vi "Configure Multi Eval Meas List Segment DMRS Type A.vi"(0 "VISA resource name":refnum<visa-resource-name>, 1 "BWP (0)":i32, 2 "Additional Position (0)":i32, 5 "Instance (1)":T2=1, 7 "Segment (1)":i32=1, 9 "CC (1)":T1=1, 11 "error in (no error)":errorcluster, 12 "Config Type (1)":i32=1, 13 "Max Length (1)":i32=1) -> (4 "VISA resource name out":refnum<visa-resource-name>, 15 "error out":errorcluster)   [LabVIEW 2020, in "Rohde&Schwarz CMWXP NR FR1 Measurement.lvlib"]
doc: "Configures the DM-RS for mapping type A. The settings apply to the <BWP> on carrier <cc> in segment <no>.\n\nAttribute:\nRSCMWXPNRFR1M_ATTR_MULTI_EVAL_MEAS_LIST_SEGMENT_DMRS_TYPE_A\n\nRemote-control command:\nCONFigure:NRSub:MEAS<i>:LIST:SEGMent<no>[:CC<cc>]:BWPart:PUSCh:DMTA"
uses:
  <instrlib>/Rohde&Schwarz CMWXP NR FR1 Measurement/Rohde&Schwarz CMWXP NR FR1 Measurement.lvlib
  <instrlib>/Rohde&Schwarz CMWXP NR FR1 Measurement/Private/_Instance.ctl
  <instrlib>/Rohde&Schwarz CMWXP NR FR1 Measurement/Private/_Carrier Component.ctl
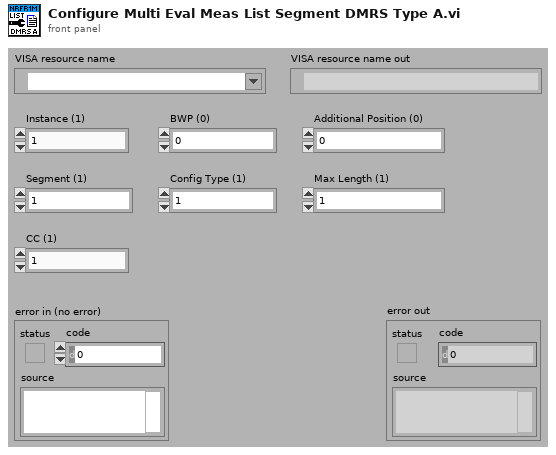
[diagram p1: front panel]
types:
  T1 = typedef "Rohde&Schwarz CMWXP NR FR1 Measurement.lvlib/_Carrier Component.ctl" = i32
  T2 = typedef "Rohde&Schwarz CMWXP NR FR1 Measurement.lvlib/_Instance.ctl" = i32
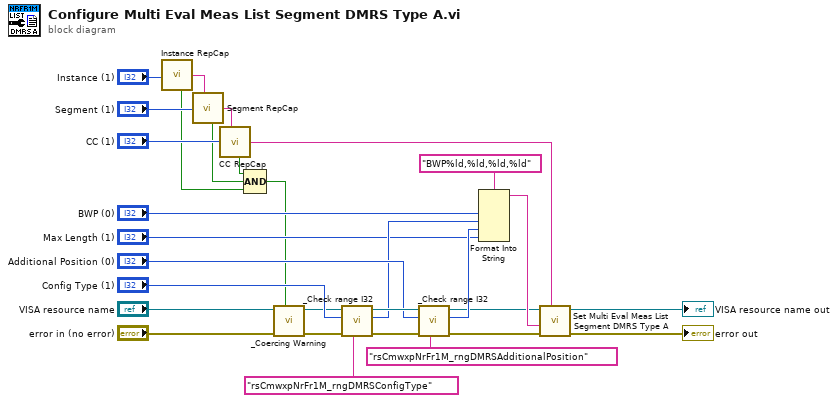
[diagram p0: block diagram]
diagram:
  n1 = call <instrlib>:"Instance RepCap.vi"("Instance In"="Instance (1)") -> ("In Range?"=w4:bool, "RepCap Identifier Out"=w15:string)  [unwired: 1 in]
  n2 = call <instrlib>:"Segment RepCap.vi"("Segment In"="Segment (1)", "RepCap String In (\"\")"=w15) -> ("In Range?"=w3:bool, "RepCap Identifier Out"=w13:string)
  n3 = call <instrlib>:"CC RepCap.vi"("CC In"="CC (1)", "RepCap String In (\"\")"=w13) -> ("In Range?"=w2:bool, "RepCap Identifier Out"=w11:string)
  n4 = Compound Arithmetic op=AND(w2, w3, w4) -> (w1:bool)
  n5 = call <instrlib>:"_Coercing Warning.vi"("In Range?"=w1, "error in (no error)"="error in (no error)", "VISA resource name"="VISA resource name") -> ("error out"=w6:errorcluster, "VISA resource name out"=w5:refnum<visa-resource-name>)  [unwired: 7 in]
  n6 = call <instrlib>:"_Check range I32.vi"("Range Table Identifier"="rsCmwxpNrFr1M_rngDMRSConfigType", "error in (no error)"=w6, "I32 Value In"="Config Type (1)", "VISA resource name"=w5) -> ("error out"=w28:errorcluster, "I32 Value Out"=w22:i32, "VISA resource name out"=w27:refnum<visa-resource-name>)  [unwired: 5 in]
  n7 = call <instrlib>:"_Check range I32.vi"("Range Table Identifier"="rsCmwxpNrFr1M_rngDMRSAdditionalPosition", "error in (no error)"=w28, "I32 Value In"="Additional Position (0)", "VISA resource name"=w27) -> ("error out"=w17:errorcluster, "I32 Value Out"=w21:i32, "VISA resource name out"=w18:refnum<visa-resource-name>)  [unwired: 5 in]
  n8 = Format Into String(format string="BWP%ld,%ld,%ld,%ld", "BWP (0)", w22, w21, "Max Length (1)") -> (resulting string=w19:string)  [unwired: 2 in, 1 out]
  n9 = call "Set Multi Eval Meas List Segment DMRS Type A"("Repeated Capabilities"=w11, "error in (no error)"=w17, "Multi Eval Meas List Segment DMRS Type A ()"=w19, "instrument handle"=w18) -> ("error out"=→"error out":errorcluster, "instrument handle out"=→"VISA resource name out":refnum<visa-resource-name>)  [unwired: 6 in]
